vi "AKIP_read.vi"(8 "error in (no error)":errorcluster, 11 "VISA Refnum in":refnum<visa-resource-name>="AKIP") -> (0 "error out":errorcluster, 2 "read buffer":string, 3 "VISA Refnum out":refnum<visa-resource-name>)   [LabVIEW 2017]
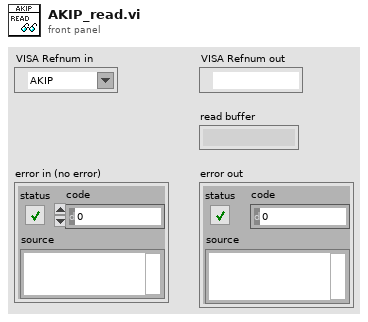
[diagram p1: front panel]
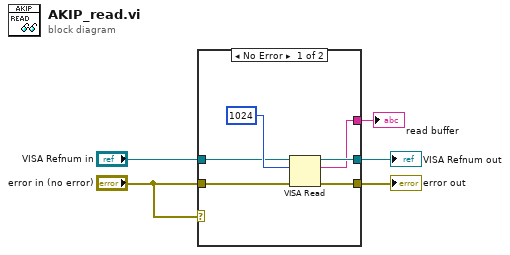
[diagram p0: block diagram]
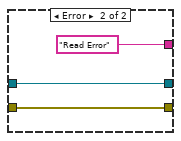
[diagram p2: hidden frame]
diagram:
  n1 = case shown="No Error" "error in (no error)" {
    tunnel: [w11 w14] -> w5
    tunnel: [w10 w13] -> w4
    tunnel: "error in (no error)" -> [w8 w13]
    tunnel: "VISA Refnum in" -> [w7 w14]
    tunnel: [w6 "Read Error" ("read buffer")] -> w2
    frame No Error {
      n2 = VISA Read(VISA resource name=w7, byte count=u32 1024, error in (no error)=w8) -> (VISA resource name out=w11:refnum<visa-resource-name>, read buffer=w6:string, error out=w10:errorcluster)  [unwired: 1 out]
    }
    frame Error {
    }
  }
  "VISA Refnum out" <- w5
  "error out" <- w4
  "read buffer" <- w2
